vi "Variant Types Equal.vi"(8 "error in (no error)":errorcluster, 10 "Type":variant, 11 "Type to Test":variant) -> (0 "error out":errorcluster, 3 "Same Type":bool)   [LabVIEW 2012, in "Scripting Tools.lvlib" / "XNode Support.lvlib"]
uses:
  XNode Support.lvlib
  <vilib>/Utility/VariantDataType/VariantType.lvlib
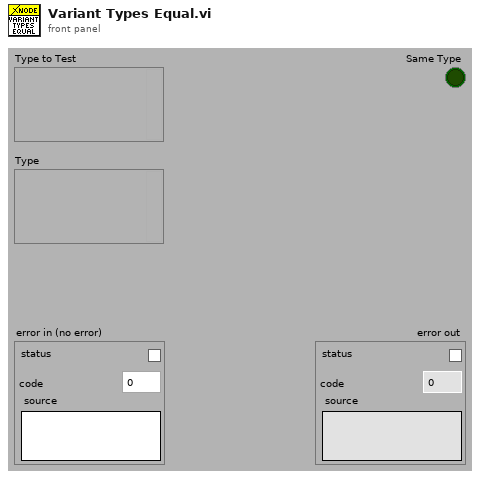
[diagram p1: front panel]
types:
  T1 = typedef "VariantType.lvlib/Type.ctl" = enum8{"Invalid Type", "Void", "I8", "I16", "I32", "I64", "U8", "U16", "U32", "U64", "Single Float", "Double Float", "Extended Float", "Single Complex", "Double Complex", "Extended Complex", "Enum U8", "Enum U16", "Enum U32", "Enum U64", "Single Float With Unit", "Double Float With Unit", "Extended Float With Unit", "Single Complex with Unit", "Double Complex with Unit", "Extended Complex with Unit", "Boolean", "String", "Path", "Picture", "Tag", "Array", "Cluster", "Variant", "LV Variant", "Waveform", "Timestamp", "Digital Waveform", "Digital Data", "ExpressData", "Refnum", "External Data", "VI", "Poly VI", "LabVIEW Class Instance", "Fixed Point"}
  T2 = typedef "VariantType.lvlib/RefnumType.ctl" = enum16{"NotARefnum", "UnknownRefnum", "Generic", "Datalog", "ByteStream", "Device", "Occurence", "TCPNetConnection", "Auto", "Menu", "Imaq", "Hardware", "DataSocket", "Visa", "IVI", "UDPNetConnection", "Notifier", "Queue", "Irda", "EventReg", "DotNet", "UserEvent", "Callback", "UNUSED_EMPTY_POSITION", "BlueToothNetConnection", "LVObjApp", "LVObjVI", "LVObjUnknown", "GenericClass", "UserDefinedRefnumTag", "DataValue", "RT FIFO", "TDMS File"}
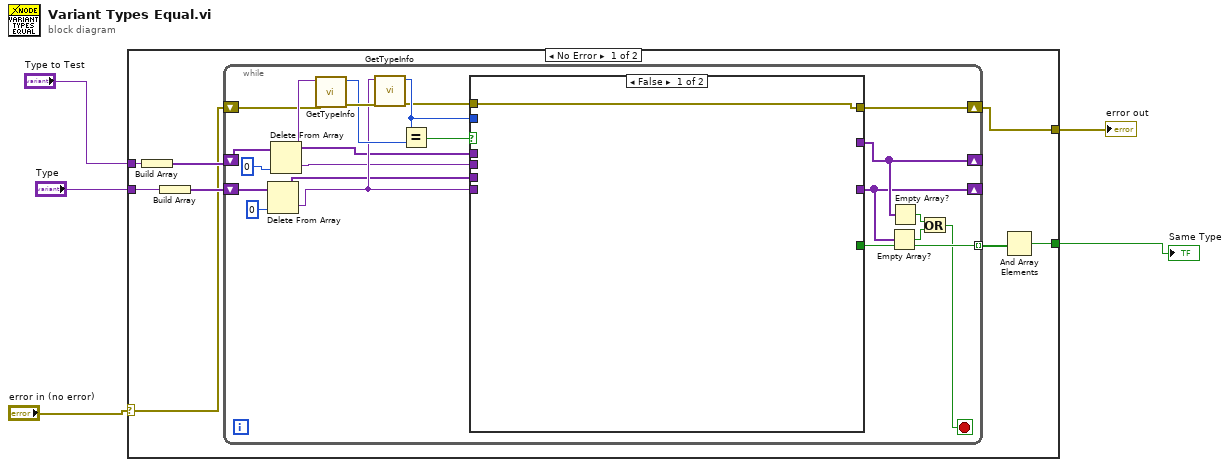
[diagram p0: block diagram]
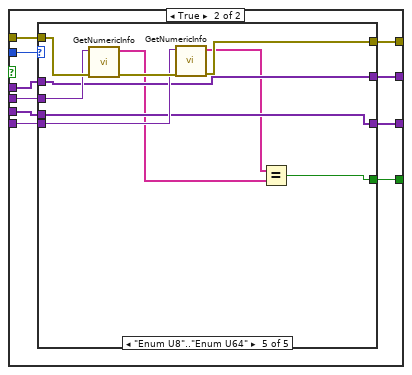
[diagram p2: hidden frame]
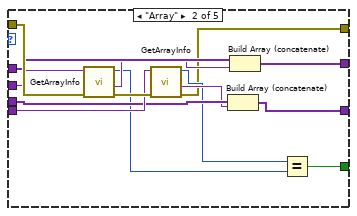
[diagram p4: hidden frame]
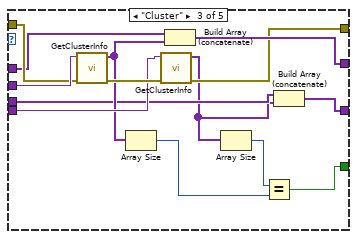
[diagram p5: hidden frame]
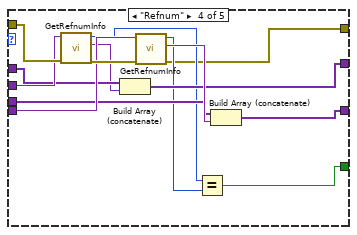
[diagram p6: hidden frame]
diagram:
  n1 = case shown="No Error" "error in (no error)" {
    selector: "error in (no error)" -> [w9 w101]
    tunnel: "Type to Test" -> [w13 _]
    tunnel: "Type" -> [w12 _]
    tunnel: [w8 w101] -> w2
    tunnel: [w6 _] -> w1
    frame No Error {
      n2 = Build Array(w13) -> (w11:variant[])
      n3 = Build Array(w12) -> (w10:variant[])
      n4 = while {
        shift-right: [w18] -> _
        shift-left: w11 -> [w34]
        shift-right: [w17] -> _
        shift-left: w10 -> [w28]
        tunnel: [w21] -> w7 mode=indexing
        shift-right: [w20] -> w8
        shift-left: w9 -> [w19]
        stop <- w14 stop-if-true
        n5 = Delete From Array(array=w28, index=0) -> (deleted portion=w25:variant, array with subset deleted=w23:variant[])  [unwired: 1 in]
        n6 = Delete From Array(array=w34, index=0) -> (deleted portion=w24:variant, array with subset deleted=w22:variant[])  [unwired: 1 in]
        n7 = call <vilib>:"GetTypeInfo.vi"("error in (no error)"=w19, "Variant"=w24) -> ("error out"=w33:errorcluster, "Type Enum"=w32:T1)  [unwired: 8 out]
        n8 = call <vilib>:"GetTypeInfo.vi"("error in (no error)"=w33, "Variant"=w25) -> ("error out"=w29:errorcluster, "Type Enum"=w30:T1)  [unwired: 8 out]
        n9 = Equal?(x=w30, y=w32) -> (x = y?=w31:bool)
        n10 = case shown="False" w31 {
          tunnel: w30 -> [_ w45]
          tunnel: w29 -> [w35 w44]
          tunnel: w25 -> [_ w43]
          tunnel: w24 -> [_ w42]
          tunnel: w23 -> [_ w41]
          tunnel: w22 -> [_ w40]
          tunnel: [_ w39] -> w18
          tunnel: [_ w38] -> w17
          tunnel: [_ w37] -> w21
          tunnel: [w35 w36] -> w20
          frame False {
          }
          frame True {
            n11 = case shown="\"Enum U8\"..\"Enum U64\"" w45 {
              tunnel: w44 -> [w46 w62 w75 w90 w100]
              tunnel: w43 -> [_ w59 w73 w87 w97]
              tunnel: w42 -> [_ w61 w76 w89 w99]
              tunnel: w41 -> [w48 w56 w68 w83 w94]
              tunnel: w40 -> [w47 w58 w72 w86 w96]
              tunnel: [w47 w54 w70 w82 w96] -> w39
              tunnel: [w48 w53 w66 w81 w94] -> w38
              tunnel: [_ w50 w63 w78 w91] -> w37
              tunnel: [w46 w49 w69 w77 w95] -> w36
              frame "Invalid Type", Default {
              }
              frame "Array" {
                n12 = call <vilib>:"GetArrayInfo.vi"("error in (no error)"=w62, "Variant"=w61) -> ("error out"=w60:errorcluster, "ArrayElement"=w57:variant, "NDims"=w51:i32)  [unwired: 7 out]
                n13 = call <vilib>:"GetArrayInfo.vi"("error in (no error)"=w60, "Variant"=w59) -> ("error out"=w49:errorcluster, "ArrayElement"=w55:variant, "NDims"=w52:i32)  [unwired: 7 out]
                n14 = Build Array (concatenate)(w56, w55) -> (w53:variant[])
                n15 = Build Array (concatenate)(w58, w57) -> (w54:variant[])
                n16 = Equal?(x=w52, y=w51) -> (x = y?=w50:bool)
              }
              frame "Cluster" {
                n17 = call <vilib>:"GetClusterInfo.vi"("error in (no error)"=w75, "Variant"=w76) -> ("error out"=w74:errorcluster, "Cluster Elements"=w71:variant[])  [unwired: 8 out]
                n18 = Array Size(array=w71) -> (size(s)=w64:i32)
                n19 = call <vilib>:"GetClusterInfo.vi"("error in (no error)"=w74, "Variant"=w73) -> ("error out"=w69:errorcluster, "Cluster Elements"=w67:variant[])  [unwired: 8 out]
                n20 = Build Array (concatenate)(w72, w71) -> (w70:variant[])
                n21 = Array Size(array=w67) -> (size(s)=w65:i32)
                n22 = Equal?(x=w65, y=w64) -> (x = y?=w63:bool)
                n23 = Build Array (concatenate)(w68, w67) -> (w66:variant[])
              }
              frame "Refnum" {
                n24 = call <vilib>:"GetRefnumInfo.vi"("error in (no error)"=w90, "Variant"=w89) -> ("error out"=w88:errorcluster, "StrictType"=w85:variant, "ReferenceType"=w80:T2)  [unwired: 7 out]
                n25 = Build Array (concatenate)(w86, w85) -> (w82:variant[])
                n26 = call <vilib>:"GetRefnumInfo.vi"("error in (no error)"=w88, "Variant"=w87) -> ("error out"=w77:errorcluster, "StrictType"=w84:variant, "ReferenceType"=w79:T2)  [unwired: 7 out]
                n27 = Equal?(x=w80, y=w79) -> (x = y?=w78:bool)
                n28 = Build Array (concatenate)(w83, w84) -> (w81:variant[])
              }
              frame "Enum U8".."Enum U64" {
                n29 = call <vilib>:"GetNumericInfo.vi"("error in (no error)"=w100, "Variant"=w99) -> ("error out"=w98:errorcluster, "EnumNames"=w92:string[])  [unwired: 8 out]
                n30 = call <vilib>:"GetNumericInfo.vi"("error in (no error)"=w98, "Variant"=w97) -> ("error out"=w95:errorcluster, "EnumNames"=w93:string[])  [unwired: 8 out]
                n31 = Equal?(x=w93, y=w92) -> (x = y?=w91:bool)
              }
            }
          }
        }
        n32 = Empty Array?(array=w17) -> (empty?=w15:bool)
        n33 = Empty Array?(array=w18) -> (empty?=w16:bool)
        n34 = Or(x=w16, y=w15) -> (x .or. y?=w14:bool)
      }
      n35 = And Array Elements(Boolean array=w7) -> (logical AND=w6:bool)
    }
    frame Error {
    }
  }
  "error out" <- w2
  "Same Type" <- w1
